vi "Generate Chessboard Image Data (Radon).vi"(7 "Add Marker (Default: False)":bool, 8 "error in (no error)":errorcluster, 10 "Chessboard Corners Info":T3, 11 "Target Size":T2) -> (0 "error out":errorcluster, 3 "Chessboard Image Data":u8[][](array[numeric]) format="%.0x")   [LabVIEW 2020, in "feature_detection.lvlib"]
doc: "Generate a chessboard for use with the Find Chessboard Corners Function and Camera Calibration."
uses:
  feature_detection.lvlib
  Chessboard Corner Info.ctl
  common/Image Size (Integer).ctl
  common/Image Point (Integer).ctl
  ChessboardSquareLocation.ctl
  Chessboard Semi Circle Square Type.ctl
  Chessboard Teardrop Corner Type.ctl
  e7f4303d-582b-4721-b29a-aa63d9231187.vi
  <vilib>/picture/picture.llb/Draw Oval.vi
  <vilib>/picture/pictutil.llb/Picture to Pixmap.vi
  <vilib>/picture/pixmap.llb/Unflatten Pixmap.vi
  <vilib>/Comparison/Equal/Equal Functor/Equal Functor.lvclass
  common/common.lvlib
panel:
  out "Origin Marker Square":T1
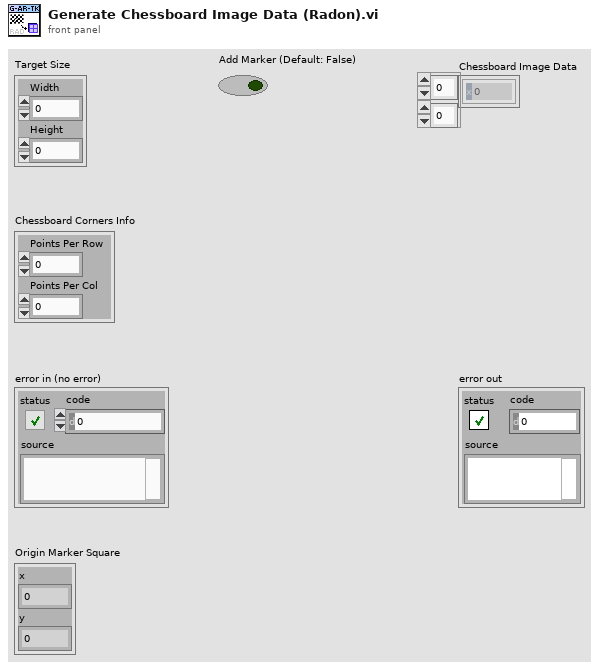
[diagram p1: front panel]
types:
  T1 = typedef "common.lvlib/Image Point (Integer).ctl" = cluster{"x":i32, "y":i32}
  T2 = typedef "common.lvlib/Image Size (Integer).ctl" = cluster{"Width":u16, "Height":u16}
  T3 = typedef "feature_detection.lvlib/Chessboard Corner Info.ctl" = cluster{"Points Per Row":u8, "Points Per Col":u8}
  T4 = typedef "feature_detection.lvlib/ChessboardSquareLocation.ctl" = enum16{"Top Left Corner", "Top Row", "Top Right Corner ", "Left Col", "Right Col", "Bottom Left Corner", "Bottom Row", "Bottom Right Corner", "Other"}
  T5 = map{cluster{"First Row":bool, "Last Row":bool, "First Col":bool, "Last Col":bool}, T4}
  T6 = cluster{"Points Per Row":i32, "Points Per Col":i32}
  T7 = cluster{"Points Per Row":i32, "Points Per Col":i32}[]
  T8 = cluster{"First Row":bool, "Last Row":bool, "First Col":bool, "Last Col":bool}
  T9 = cluster{"left":i32, "top":i32, "right":i32, "bottom":i32}
  T10 = typedef "feature_detection.lvlib/Chessboard Semi Circle Square Type.ctl" = enum16{"Top", "Left", "Right", "Bottom"}
  T11 = typedef "feature_detection.lvlib/Chessboard Teardrop Corner Type.ctl" = enum16{"Top Left", "Top Right", "Bottom Left", "Bottom Right"}
  T12 = cluster{"Width":i16, "Style":enum32{"Solid", "Dash", "Dot", "DashDot", "DashDotDot"}}
  T13 = cluster{"left":i16, "top":i16, "right":i16, "bottom":i16}
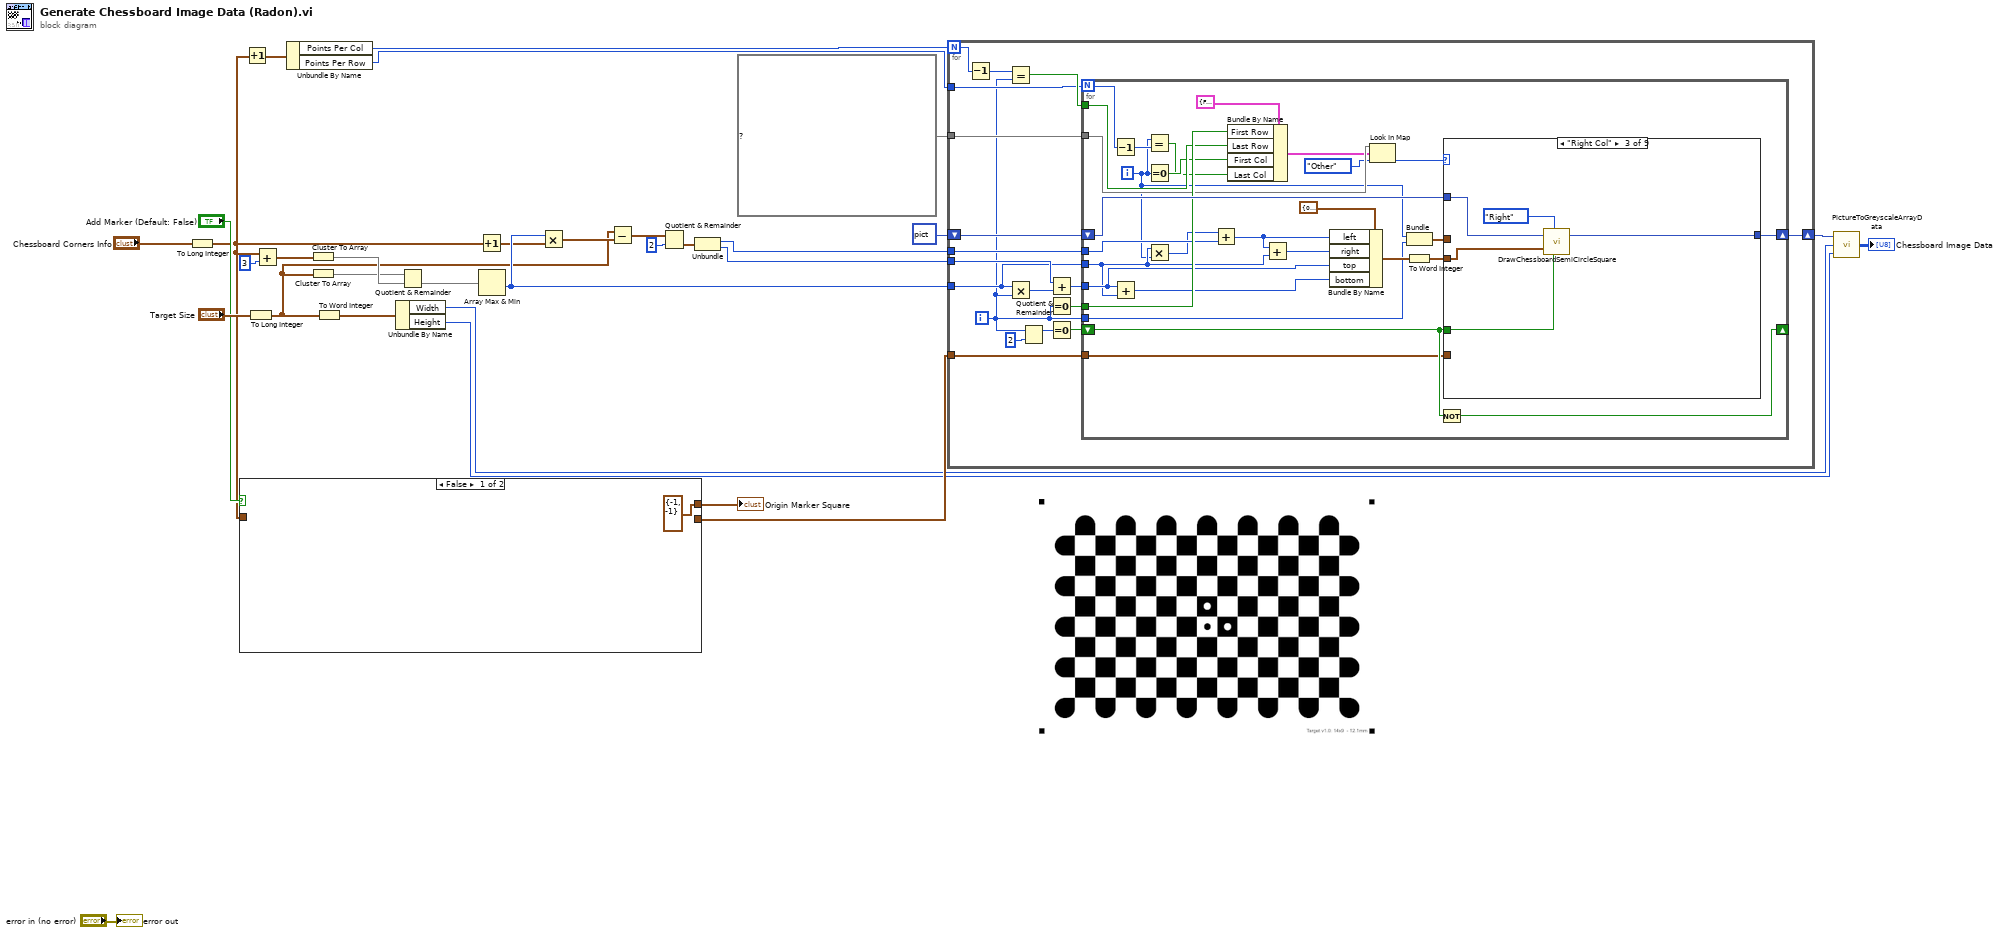
[diagram p0: block diagram]
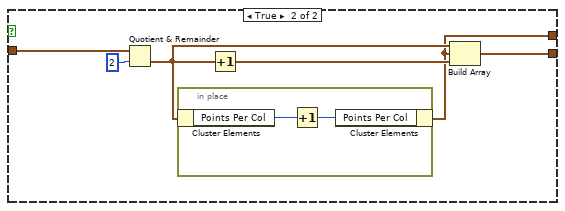
[diagram p2: hidden frame]
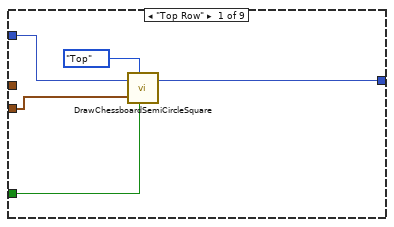
[diagram p3: hidden frame]
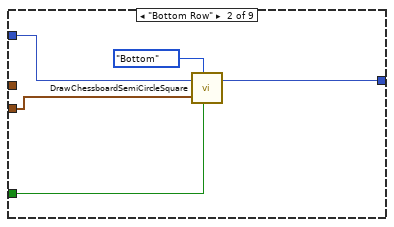
[diagram p4: hidden frame]
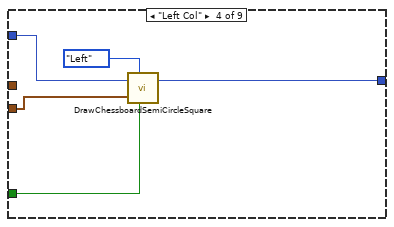
[diagram p5: hidden frame]
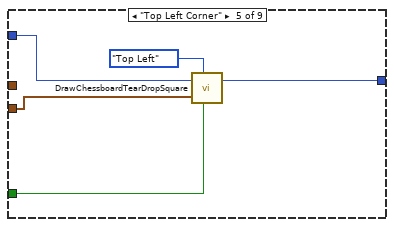
[diagram p6: hidden frame]
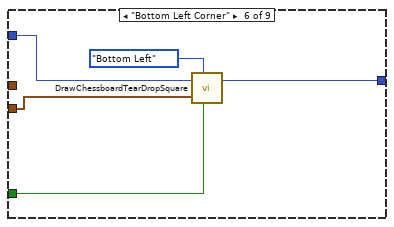
[diagram p7: hidden frame]
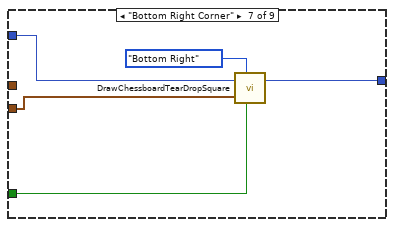
[diagram p8: hidden frame]
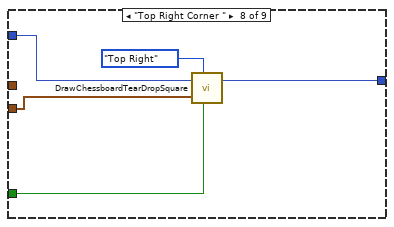
[diagram p9: hidden frame]
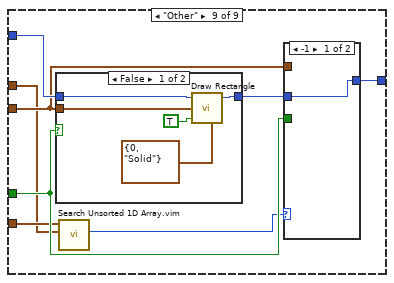
[diagram p10: hidden frame]
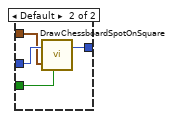
[diagram p11: hidden frame]
diagram:
  n1 = To Long Integer(number="Chessboard Corners Info") -> (32bit integer=w5:T6)
  n2 = case shown="False" "Add Marker (Default: False)" {
    tunnel: w5 -> [_ w38]
    tunnel: [_ w36] -> w6
    tunnel: [T6 {"Points Per Row"=-1, "Points Per Col"=-1} w33] -> w4
    frame False {
    }
    frame True {
      n3 = Quotient & Remainder(x=w38, y=2) -> (floor(x/y)=w35:T6)  [unwired: 1 out]
      n4 = in-place {
        n5 = in-place-cluster #1(w35) -> ("Points Per Col"=w40:i32)
        n6 = Increment(x=w40) -> (x+1=w39:i32)
        n7 = in-place-cluster #1("Points Per Col"=w39) -> (w33:T6)
      }
      n8 = Increment(x=w35) -> (x+1=w34:T6)
      n9 = Build Array(w35, w33, w34) -> (w36:T7)
    }
  }
  "Origin Marker Square" <- w4
  n10 = Increment(x=w5) -> (x+1=w8:T6)
  n11 = To Long Integer(number="Target Size") -> (32bit integer=w15:cluster{"Width":i32, "Height":i32})
  n12 = Add(x=w5, y=3) -> (x+y=w24:T6)
  n13 = Unbundle By Name(w8) -> ("Points Per Col"=w27:i32, "Points Per Row"=w9:i32)
  n14 = Cluster To Array(cluster=w24) -> (array=w17:i32[])
  n15 = Cluster To Array(cluster=w15) -> (array=w16:i32[])
  n16 = To Word Integer(number=w15) -> (16bit integer=w23:cluster{"Width":i16, "Height":i16})
  n17 = Unbundle By Name(w23) -> ("Width"=w2:i16, "Height"=w1:i16)
  n18 = Quotient & Remainder(x=w16, y=w17) -> (floor(x/y)=w29:i32[])  [unwired: 1 out]
  n19 = Increment(x=w5) -> (x+1=w18:T6)
  n20 = Array Max & Min(array=w29) -> (min value=w25:i32)  [unwired: 3 out]
  n21 = Multiply(x=w25, y=w18) -> (x*y=w22:T6)
  n22 = Subtract(x=w15, y=w22) -> (x-y=w21:cluster{i32, i32})
  n23 = Quotient & Remainder(x=w21, y=2) -> (floor(x/y)=w14:cluster{i32, i32})  [unwired: 1 out]
  n24 = Unbundle(w14) -> (w20:i32, w19:i32)
  n25 = for {
    N: w27 -> [w53]
    shift-right: [w57] -> w26
    shift-left: picture data[5B] ("picture") -> [w58]
    tunnel: w25 -> [w46]
    tunnel: w20 -> [w50]
    tunnel: w19 -> [w49]
    tunnel: T5 {{"First Row"=FALSE, "Last Row"=FALSE, "First Col"=FALSE, "Last Col"=TRUE}=enum."Right Col", {"First Row"=FALSE, "Last Row"=FALSE, "First Col"=TRUE, "Last Col"=FALSE}=enum."Left Col", {"First Row"=FALSE, "Last Row"=TRUE, "First Col"=FALSE, "Last Col"=FALSE}=enum."Bottom Row", {"First Row"=FALSE, "Last Row"=TRUE, "First Col"=FALSE, "Last Col"=TRUE}=enum."Bottom Right Corner", {"First Row"=FALSE, "Last Row"=TRUE, "First Col"=TRUE, "Last Col"=FALSE}=enum."Bottom Left Corner", {"First Row"=TRUE, "Last Row"=FALSE, "First Col"=FALSE, "Last Col"=FALSE}=enum."Top Row", {"First Row"=TRUE, "Last Row"=FALSE, "First Col"=FALSE, "Last Col"=TRUE}=enum."Top Right Corner ", {"First Row"=TRUE, "Last Row"=FALSE, "First Col"=TRUE, "Last Col"=FALSE}=enum."Top Left Corner"} ("Map") -> [w54]
    tunnel: w9 -> [w51]
    tunnel: w6 -> [w42]
    i -> [w41]
    n26 = Decrement(x=w53) -> (x-1=w52:i32)
    n27 = Equal?(x=w52, y=w41) -> (x = y?=w55:bool)
    n28 = Multiply(x=w46, y=w41) -> (x*y=w47:i32)
    n29 = Quotient & Remainder(x=w41, y=2) -> (x-y*floor(x/y)=w44:i32)  [unwired: 1 out]
    n30 = Add(x=w49, y=w47) -> (x+y=w48:i32)
    n31 = Equal To 0?(x=w41) -> (x = 0?=w56:bool)
    n32 = Equal To 0?(x=w44) -> (x = 0?=w43:bool)
    n33 = for {
      N: w51 -> [w76]
      shift-right: [w85] -> w57
      shift-left: w58 -> [w87]
      tunnel: w56 -> [w81]
      tunnel: w55 -> [w80]
      tunnel: w54 -> [w79]
      tunnel: w46 -> [w66]
      tunnel: w50 -> [w69]
      tunnel: w48 -> [w68]
      shift-right: [w64] -> _
      shift-left: w43 -> [w63]
      tunnel: w42 -> [w62]
      tunnel: w41 -> [w59]
      i -> [w60]
      n34 = Decrement(x=w76) -> (x-1=w75:i32)
      n35 = Add(x=w68, y=w66) -> (x+y=w73:i32)
      n36 = Equal?(x=w60, y=w75) -> (x = y?=w70:bool)
      n37 = Equal To 0?(x=w60) -> (x = 0?=w71:bool)
      n38 = Multiply(x=w66, y=w60) -> (x*y=w65:i32)
      n39 = Add(x=w65, y=w69) -> (x+y=w67:i32)
      n40 = Bundle By Name(cluster=T8 {"First Row"=FALSE, "Last Row"=FALSE, "First Col"=FALSE, "Last Col"=FALSE} ("Position"), "First Row"=w81, "Last Row"=w80, "First Col"=w71, "Last Col"=w70) -> (w78:T8)
      n41 = Add(x=w67, y=w66) -> (x+y=w74:i32)
      n42 = Bundle By Name(cluster=T9 {"left"=0, "top"=0, "right"=0, "bottom"=0} ("32bit integer"), "left"=w67, "right"=w74, "top"=w68, "bottom"=w73) -> (w86:T9)
      n43 = Look In Map(map=w79, key=w78, default value=ChessboardSquareLocation."Other") -> (value=w72:T4)  [unwired: 1 out]
      n44 = To Word Integer(number=w86) -> (16bit integer=w84:T13)
      n45 = Bundle(w60, w59) -> (w61:cluster{i32, i32})  [unwired: 1 in]
      n46 = Not(x=w63) -> (.not. x?=w64:bool)
      n47 = case shown="\"Right Col\"" w72 {
        tunnel: w87 -> [w92 w97 w102 w107 w112 w117 w122 w127 w135]
        tunnel: [w91 w96 w101 w106 w111 w116 w121 w126 w133] -> w85
        tunnel: w84 -> [w90 w95 w100 w105 w110 w115 w120 w125 w131]
        tunnel: w63 -> [w88 w93 w98 w103 w108 w113 w118 w123 w132]
        tunnel: w62 -> [_ _ _ _ _ _ _ _ w130]
        tunnel: w61 -> [_ _ _ _ _ _ _ _ w129]
        frame "Top Row" {
          n48 = call "DrawChessboardSemiCircleSquare.vi"("Bounds"=w90, "Skip"=w88, "picture in"=w92, "Semi Circle Square Type"=Chessboard_Semi_Circle_Square_Type."Top") -> ("picture out"=w91:picture)  [unwired: 3 in]
        }
        frame "Bottom Row" {
          n49 = call "DrawChessboardSemiCircleSquare.vi"("Bounds"=w95, "Skip"=w93, "picture in"=w97, "Semi Circle Square Type"=Chessboard_Semi_Circle_Square_Type."Bottom") -> ("picture out"=w96:picture)  [unwired: 3 in]
        }
        frame "Right Col" {
          n50 = call "DrawChessboardSemiCircleSquare.vi"("Bounds"=w100, "Skip"=w98, "picture in"=w102, "Semi Circle Square Type"=Chessboard_Semi_Circle_Square_Type."Right") -> ("picture out"=w101:picture)  [unwired: 3 in]
        }
        frame "Left Col" {
          n51 = call "DrawChessboardSemiCircleSquare.vi"("Bounds"=w105, "Skip"=w103, "picture in"=w107, "Semi Circle Square Type"=Chessboard_Semi_Circle_Square_Type."Left") -> ("picture out"=w106:picture)  [unwired: 3 in]
        }
        frame "Top Left Corner" {
          n52 = call "DrawChessboardTearDropSquare.vi"("Bounds"=w110, "Skip"=w108, "picture in"=w112, "Tear Drop Corner"=Chessboard_Teardrop_Corner_Type."Top Left") -> ("picture out"=w111:picture)  [unwired: 3 in]
        }
        frame "Bottom Left Corner" {
          n53 = call "DrawChessboardTearDropSquare.vi"("Bounds"=w115, "Skip"=w113, "picture in"=w117, "Tear Drop Corner"=Chessboard_Teardrop_Corner_Type."Bottom Left") -> ("picture out"=w116:picture)  [unwired: 3 in]
        }
        frame "Bottom Right Corner" {
          n54 = call "DrawChessboardTearDropSquare.vi"("Bounds"=w120, "Skip"=w118, "picture in"=w122, "Tear Drop Corner"=Chessboard_Teardrop_Corner_Type."Bottom Right") -> ("picture out"=w121:picture)  [unwired: 3 in]
        }
        frame "Top Right Corner " {
          n55 = call "DrawChessboardTearDropSquare.vi"("Bounds"=w125, "Skip"=w123, "picture in"=w127, "Tear Drop Corner"=Chessboard_Teardrop_Corner_Type."Top Right") -> ("picture out"=w126:picture)  [unwired: 3 in]
        }
        frame "Other" {
          n56 = case shown="False" w132 {
            tunnel: w135 -> [w145 w146]
            tunnel: [w144 w146] -> w134
            tunnel: w131 -> [w143 _]
            frame False {
              n57 = call <vilib>:"Draw Rectangle.vi"("picture"=w145, "rect"=w143, "fill?(F)"=TRUE, "pen"=T12 {"Width"=0, "Style"=enum."Solid"}) -> ("new picture"=w144:picture)  [unwired: 5 in]
            }
            frame True {
            }
          }
          n58 = call "Search Unsorted 1D Array.vim"("element"=w129, "unsorted 1D array"=w130) -> ("index of element"=w128:i32)  [unwired: 9 in]
          n59 = case shown="-1" w128 {
            tunnel: w134 -> [w136 w140]
            tunnel: [w136 w139] -> w133
            tunnel: w132 -> [_ w138]
            tunnel: w131 -> [_ w137]
            frame -1 {
            }
            frame Default {
              n60 = call "DrawChessboardSpotOnSquare.vi"("Bounds"=w137, "Black On White"=w138, "picture in"=w140) -> ("picture out"=w139:picture)  [unwired: 4 in]
            }
          }
        }
      }
    }
  }
  n61 = call "PictureToGreyscaleArrayData.vi"("Bottom"=w1, "Right"=w2, "Picture"=w26) -> ("Greyscale Image Data"=→"Chessboard Image Data":u8[][])  [unwired: 2 in]
  "error out" <- "error in (no error)"
